vi "Compute Clock Frequency.vi"(11 "SPI Divide Value":u8) -> (3 "SPI Clock Frequency (Hz)":dbl format="%_6f")   [LabVIEW 2014, in "SLSC configuration System Explorer.lvlib"]
uses:
  SLSC configuration System Explorer.lvlib
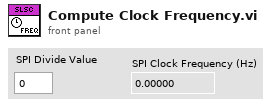
[diagram p1: front panel]
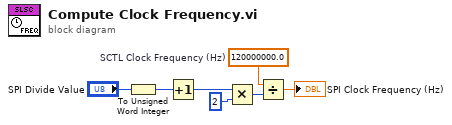
[diagram p0: block diagram]
diagram:
  w7 = 120000000.0  # SCTL Clock Frequency (Hz)
  n1 = To Unsigned Word Integer(number="SPI Divide Value") -> (unsigned 16bit integer=w1:u16)
  n2 = Increment(x=w1) -> (x+1=w5:u16)
  n3 = Multiply(x=w5, y=u16 2) -> (x*y=w3:u16)
  n4 = Divide(x=w7, y=w3) -> (x/y=→"SPI Clock Frequency (Hz)":dbl)
